vi "LINX - PmodBT2.vi"() -> ()   [LabVIEW 2014, in "LMH-LINX.lvlib"]
doc: "PmodMAXSONOR\n\nThis example demonstrates how to read the relative light sensed by the PmodALS.\n\nInstructions:\n1. Select the COM Port associated with the LINX device\n2. Select the UART Channel that the Pmod is connected to.\n3. Click the Run Arrow."
uses:
  vi.lib/MakerHub/LINX/LMH-LINX.lvlib
  vi.lib/MakerHub/LINX/Public/Sensors/Pmods/BT2/PmodBT2.lvlib
panel:
  in  "Stop Button":bool
  in  "Add <n>?":bool
  in  "Command to Send":string
  out "Reading":string
  in  "Bytes to Read":u32
  in  "Send Command":bool
  in  "Serial Port":refnum<visa-resource-name>="N/A"
  in  "UART Channel (0)":u8
  # "PmodBT2\n\nThis example demonstrates how send commands and receive transmissions from PmodBT2.\n\nInstructions:\n1. Select the COM Port associated with the LINX device\n2. Select the UART Channel that the Pmod is connected to.\n3. Enter the number of bytes you want to read on your bluetooth connection.\n4. Click the Run Arrow."
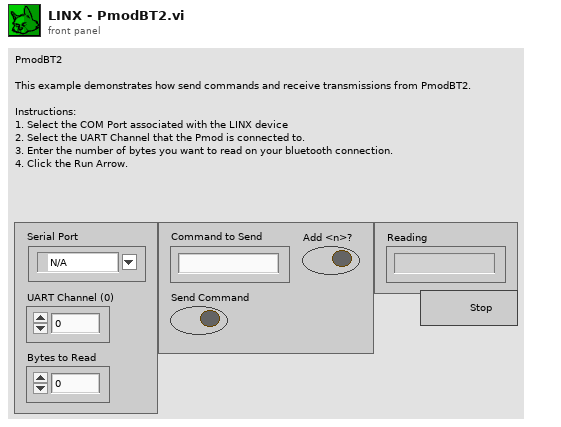
[diagram p1: front panel]
types:
  T1 = typedef "LMH-LINX.lvlib/LINX Ref.ctl" = cluster{"Platform":T2, "Interface":T3, "LINX Device Config":T4}
  T2 = typedef "LMH-LINX.lvlib/Platform.ctl" = enum16{"LINX", "myRIO"}
  T3 = typedef "LMH-LINX.lvlib/Interface.ctl" = enum16{"Serial", "TCP"}
  T4 = typedef "LMH-LINX.lvlib/Device.lvlib/LINX Device Config.ctl" = cluster{"Interface":T3, "COM Port":refnum<visa-resource-name>, "TCP Configuration":T5, "Device Family":u8, "Device ID":u8, "Device Name":string, "TCP Ref":refnum<k5>, "Channels":T6}
  T5 = typedef "LMH-LINX.lvlib/Device.lvlib/TCP Config.ctl" = cluster{"IP Address":string, "Port":u16}
  T6 = typedef "LMH-LINX.lvlib/Channels.ctl" = cluster{"DI":u8[], "DO":u8[], "AI":u8[], "AO":u8[], "PWM":u8[], "QE":u8[], "UART":u8[], "I2C 2":u8[], "SPI":u8[], "CAN":u8[], "Servo":u8[], "AI Ref (V)":dbl, "AO Ref (V)":dbl, "AO Resolution (Bits)":u8}
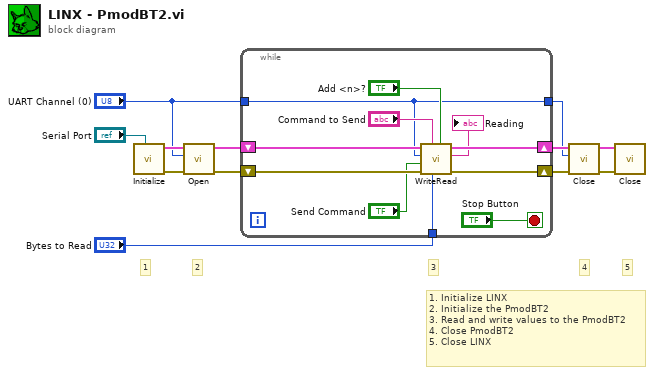
[diagram p0: block diagram]
diagram:
  # "1. Initialize LINX\n2. Initialize the PmodBT2\n3. Read and write values to the PmodBT2\n4. Close PmodBT2\n5. Close LINX"
  # "5"
  # "4"
  # "3"
  # "2"
  # "1"
  n1 = call "Initialize.vi"("Serial Port"="Serial Port") -> ("Error Out"=w12:errorcluster, "LINX Resource"=w11:T1)  [unwired: 8 in, 1 out]
  n2 = call "Open.vi"("Error In"=w12, "UART Channel (0)"="UART Channel (0)", "LINX Resource"=w11) -> ("Error Out"=w8:errorcluster, "LINX Resource"=w9:T1)  [unwired: 7 in]
  n3 = while {
    tunnel: "UART Channel (0)" -> [w13]
    tunnel: "Bytes to Read" -> [w20]
    shift-right: [w18] -> w4
    shift-left: w9 -> [w23]
    shift-right: [w19] -> w5
    shift-left: w8 -> [w22]
    tunnel: [w13] -> w1
    stop <- "Stop Button" stop-if-true
    n4 = call "WriteRead.vi"("Add <n>?"="Add <n>?", "Bytes to Read"=w20, "Command to Send"="Command to Send", "Error In"=w22, "Send Command"="Send Command", "UART Channel (0)"=w13, "LINX Resource"=w23) -> ("Error Out"=w19:errorcluster, "Data"=→"Reading":string, "LINX Resource"=w18:T1)  [unwired: 2 in]
  }
  n5 = call "Close.vi"("Error In"=w5, "UART Channel (0)"=w1, "LINX Resource"=w4) -> ("Error Out"=w2:errorcluster, "LINX Resource"=w3:T1)  [unwired: 7 in]
  n6 = call "Close.vi"("Error In"=w2, "LINX Resource"=w3) -> ()  [unwired: 9 in, 1 out]
